vi "getActorParametersJson.vi"(8 "error":errorcluster, 9 "param_list":string, 10 "axis":i32, 11 "connection ID":refnum<k5>) -> (0 "error out":errorcluster, 1 "parameters":string, 2 "axis_out":i32, 3 "connection ID out":refnum<k5>)   [LabVIEW 2016, in "amc_api.lvlib"]
doc: "This function reads the current values of the given set of actor-parameters and retuns them as key-value-pairs in a json-string"
uses:
  amc_api.lvlib
panel:
  out "jsonRespIn":string
  out "JSON-response":string="{\"jsonrpc\":\"2.0\",\"method\":\"\",\"params\":[5,1.245,true,\"name\"],\"id\":\"1\"}"
  out "JSON request":string
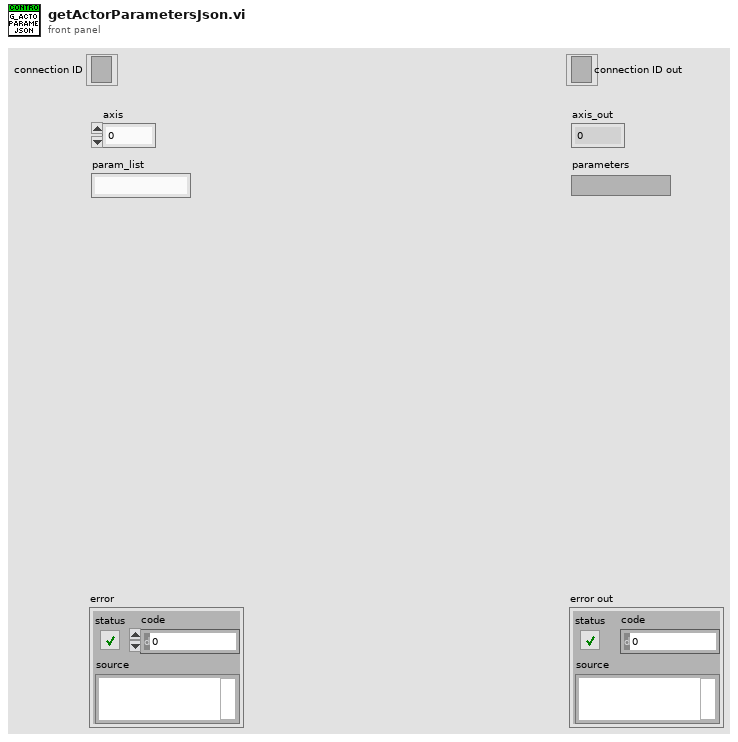
[diagram p1: front panel]
types:
  T1 = cluster{"jsonrpc":string, "method":string, "params":string[], "id":string, "api":i32, "pid":string}
  T2 = enum16{"Standard", "Buffered", "CRLF", "Immediate"}
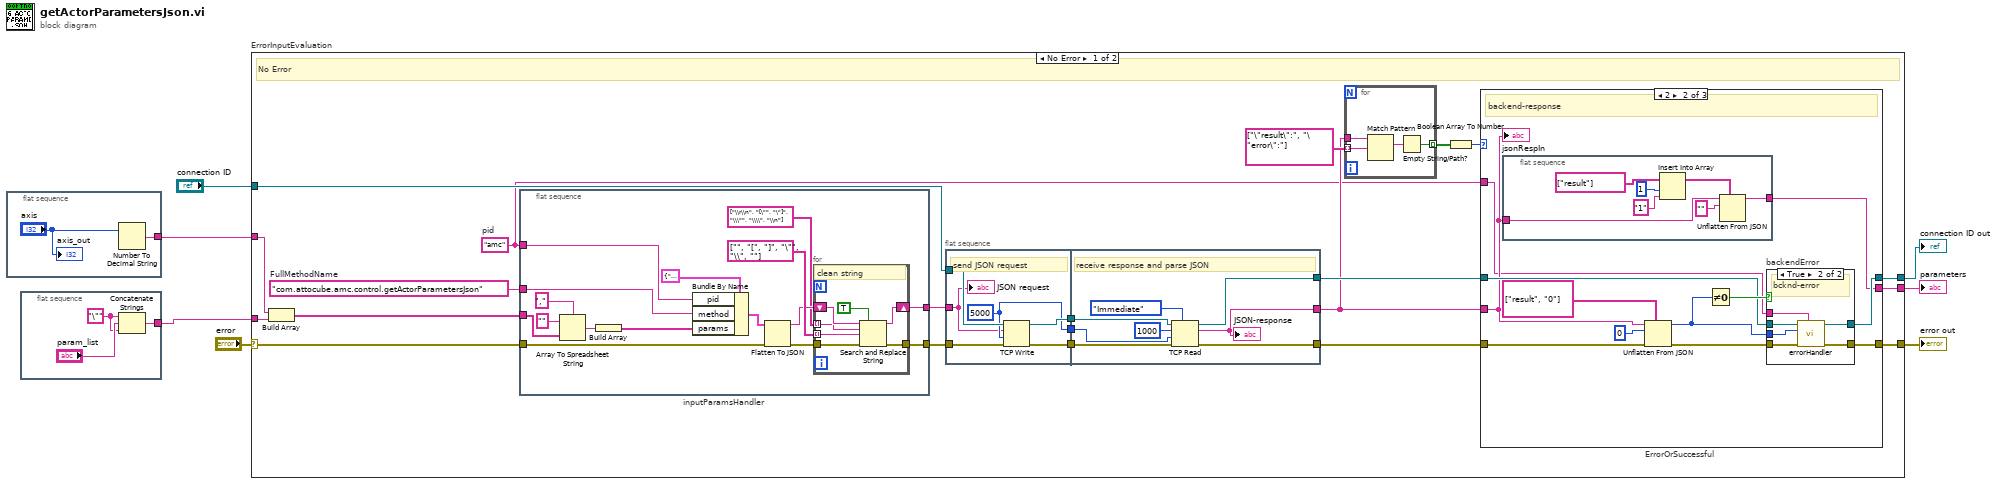
[diagram p0: block diagram]
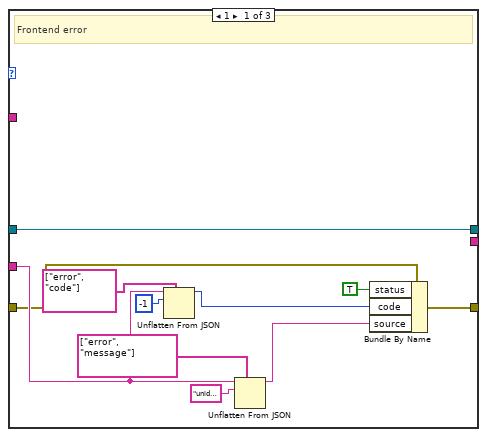
[diagram p2: hidden frame]
diagram:
  n1 = flat-sequence "in_axis" {
    tunnel: [w9] -> w3
    frame #0 {
      n2 = Number To Decimal String(number="axis") -> (decimal integer string=w9:string)  [unwired: 1 in]
      "axis_out" <- "axis"
    }
  }
  n3 = flat-sequence "in_string" {
    tunnel: [w11] -> w2
    frame #0 {
      w10 = "\"" ("string")
      n4 = Concatenate Strings(w10, "param_list", w10) -> (w11:string)
    }
  }
  n5 = case "ErrorInputEvaluation" shown="No Error" "error" {
    selector: "error" -> [w20 w115]
    tunnel: "connection ID" -> [w30 w116]
    tunnel: [w22 w115] -> w6
    tunnel: [w23 w116] -> w5
    tunnel: w3 -> [w15 _]
    tunnel: w2 -> [w14 _]
    tunnel: [w13 _] -> w1
    frame No Error {
      w16 = "amc"  # pid
      w21 = "com.attocube.amc.control.getActorParametersJson"  # FullMethodName
      # "No Error"
      n6 = Build Array ("ParametersArrayString")(w15, w14) -> (w19:string[])
      n7 = flat-sequence "inputParamsHandler" {
        tunnel: [w39] -> w18
        tunnel: w19 -> [w45]
        tunnel: w20 -> [w44]
        tunnel: [w41] -> w17
        tunnel: w21 -> [w35]
        tunnel: w16 -> [w34]
        frame #0 {
          n8 = Array To Spreadsheet String(delimiter (Tab)=",", array=w45, 3:"" ("format string")) -> (spreadsheet string=w47:string)
          n9 = Build Array "Build Array"(w47) -> (w36:string[])
          n10 = Bundle By Name(cluster=T1 {"jsonrpc"="2.0", "method"="com.attocube.amc.res.setRESReadOutFreq", "params"=[], "id"="1", "api"=2, "pid"=""}, "pid"=w34, "method"=w35, "params"=w36) -> (w46:T1)
          n11 = Flatten To JSON(anything=w46, error in (no error)=w44) -> (JSON string=w40:string, 11:w42:errorcluster)  [unwired: 1 in]
          n12 = for {
            tunnel: string[] ["\\r\\n", "[\"", "\"]", "\\\"", "\\\\", "\\n"] ("search string") -> [w53] mode=indexing
            tunnel: string[] ["", "[", "]", "\"", "\\", ""] ("replace string (\"\")") -> [w52] mode=indexing
            shift-right: [w55] -> w39
            shift-left: w40 -> [w54]
            tunnel: w42 -> [w51]
            tunnel: [w50] -> w41
            # "clean string"
            n13 = Search and Replace String(replace all?=TRUE ("replace all? (F)"), input string=w54, search string=w53, replace string=w52, error in=w51) -> (result string=w55:string, error out=w50:errorcluster)  [unwired: 3 in, 2 out]
          }
        }
      }
      n14 = flat-sequence {
        tunnel: w30 -> [w106]
        tunnel: [w104] -> w33
        tunnel: [w105] -> w32
        tunnel: w17 -> [w101]
        tunnel: [w103] -> w31
        tunnel: w18 -> [w102]
        tunnel: [w110] -> w26
        tunnel: w33 -> [w112]
        tunnel: w32 -> [w111]
        tunnel: [w108] -> w25
        tunnel: w31 -> [w109]
        tunnel: [w107] -> w24
        frame #0 {
          w103 = 5000 ("timeout ms (25000)")
          # "send JSON request"
          n15 = TCP Write(connection ID=w106, data in=w102, error in (no error)=w101, 9:w103) -> (connection ID out=w104:refnum<k5>, error out=w105:errorcluster)  [unwired: 1 out]
          "JSON request" <- w102
        }
        frame #1 {
          # "receive response and parse JSON"
          n16 = TCP Read(connection ID=w112, bytes to read=1000, error in (no error)=w111, 7:T2."Immediate" ("mode (standard)"), 9:w109) -> (connection ID out=w110:refnum<k5>, data out=w107:string, error out=w108:errorcluster)
          "JSON-response" <- w107
        }
      }
      n17 = for {
        tunnel: string[] ["\"result\":", "\"error\":"] ("path") -> [w59] mode=indexing
        tunnel: [w57] -> w28 mode=indexing
        tunnel: w24 -> [w60]
        n18 = Match Pattern(string=w60, regular expression=w59) -> (match substring=w58:string)  [unwired: 1 in, 3 out]
        n19 = Empty String/Path?(string/path=w58) -> (empty?=w57:bool)
      }
      n20 = Boolean Array To Number(Boolean array=w28) -> (number=w27:u32)
      n21 = case "ErrorOrSuccessful" shown="2" w27 {
        tunnel: w24 -> [w63 w74 _]
        tunnel: w26 -> [w61 w77 w100]
        tunnel: [w61 w76 w100] -> w23
        tunnel: [w64 w75 w99] -> w22
        tunnel: w25 -> [w62 w78 w99]
        tunnel: w16 -> [_ w73 _]
        tunnel: [_ w72 _] -> w13
        frame 1 {
          # "Frontend error"
          n22 = Unflatten From JSON(path=string[] ["error", "code"], JSON string=w63, type and defaults=-1) -> (value=w70:i32)  [unwired: 4 in, 1 out]
          n23 = Unflatten From JSON(path=string[] ["error", "message"], JSON string=w63, type and defaults="unidentified error") -> (value=w71:string)  [unwired: 4 in, 1 out]
          n24 = Bundle By Name(cluster=w62, "status"=TRUE, "code"=w70, "source"=w71) -> (w64:errorcluster)
        }
        frame 2 {
          # "backend-response"
          n25 = flat-sequence "out_string" {
            tunnel: w74 -> [w90]
            tunnel: [w84] -> w72
            frame #0 {
              n26 = Insert Into Array(array=string[] ["result"] ("path"), index=1, new element="1" ("idx")) -> (w87:string[])
              n27 = Unflatten From JSON(path=w87, JSON string=w90, type and defaults="") -> (value=w84:string)  [unwired: 4 in, 1 out]
            }
          }
          n28 = Unflatten From JSON(path=string[] ["result", "0"], JSON string=w74, type and defaults=0, error in (no error)=w78) -> (value=w83:i32, error out=w81:errorcluster)  [unwired: 3 in]
          n29 = Not Equal To 0?(x=w83) -> (x != 0?=w82:bool)
          n30 = case "backendError" shown="True" w82 {
            tunnel: w83 -> [_ w98]
            tunnel: w81 -> [w92 w97]
            tunnel: [w91 w96] -> w76
            tunnel: [w92 w95] -> w75
            tunnel: w77 -> [w91 w94]
            tunnel: w73 -> [_ w93]
            frame False {
              # "successful"
            }
            frame True {
              # "bcknd-error"
              n31 = call "errorHandler.vi"("pid"=w93, "error in"=w97, "errNbr"=w98, "connection ID"=w94) -> ("error out 2"=w95:errorcluster, "connection ID out"=w96:refnum<k5>)  [unwired: 6 in]
            }
          }
          "jsonRespIn" <- w74
        }
        frame Default {
          # "NoResponse"
        }
      }
    }
    frame Error {
      # "Error"
    }
  }
  "error out" <- w6
  "connection ID out" <- w5
  "parameters" <- w1
